vi "Set Dashboard LEDs.vi"(8 "Display code":u8, 11 "FPGA VI Reference in":T1) -> (3 "FPGA VI Reference out":T1)   [LabVIEW 2009]
uses:
  TypeDefs/Sensor TypeDefs/FPGA Main ref.ctl
  <vilib>/rvi/interface/nirviReadWriteControl/nirviReadWriteControl.xnode
  FPGA Bitfiles/Q_IGVC_2010.lvproj_FPGA Target_FPGA_MAIN.vi.lvbitx
  <vilib>/Utility/error.llb/Error Cluster From Error Code.vi
  <vilib>/rvi/errors/niLvFpgaAdjustHostInterfaceError.vi
  <vilib>/rvi/interface/common/niFpgaNodeNameForErrorReporting.ctl
  <vilib>/rvi/errors/niLvFpgaWhatHappensToTopLevelVI.ctl
  NiRioSrv.dll
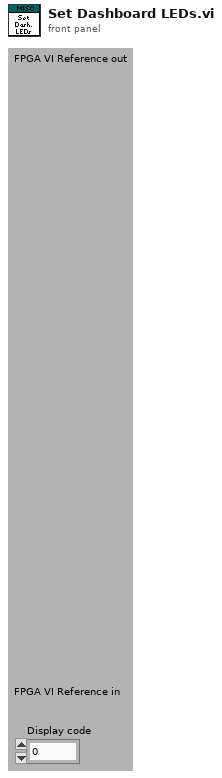
[diagram p1: front panel]
types:
  T1 = typedef "FPGA Main ref.ctl" = refnum<k20>
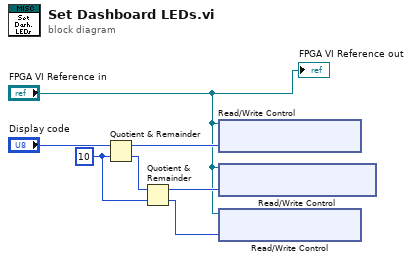
[diagram p0: block diagram]
diagram:
  w6 = u8 10 ("y")
  n1 = Quotient & Remainder(x="Display code", y=w6) -> (x-y*floor(x/y)=w5:u8, floor(x/y)=w7:u8)
  n2 = Quotient & Remainder(x=w7, y=w6) -> (x-y*floor(x/y)=w4:u8, floor(x/y)=w3:u8)
  n3 = xnode "Read/Write Control"("FPGA VI Reference In"="FPGA VI Reference in", "GO LED ON/OFF/BLINK"=w5) -> ()  [unwired: 1 in, 2 out]
  n4 = xnode "Read/Write Control"("FPGA VI Reference In"="FPGA VI Reference in", "Safety LED ON/OFF/BLINK"=w4) -> ()  [unwired: 1 in, 2 out]
  n5 = xnode "Read/Write Control"("FPGA VI Reference In"="FPGA VI Reference in", "Init LED ON/OFF/BLINK"=w3) -> ()  [unwired: 1 in, 2 out]
  "FPGA VI Reference out" <- "FPGA VI Reference in"
